vi "get channels.vi"(11 "module configuration in":refnum<class "PID Module configuration.lvclass">) -> (2 "channels":refnum<class "TBM channel.lvclass">[](array[class]), 3 "module configuration out":refnum<class "PID Module configuration.lvclass">)   [LabVIEW 2013, in "PID Module configuration.lvclass"]
doc: "Returns all channels used by a module."
uses:
  PID Module configuration.lvclass
  <vilib>/NI/Tag Bus Module Framework/module configuration/TBM module configuration.lvclass
  <vilib>/NI/Tag Bus Module Framework/channel/TBM channel.lvclass
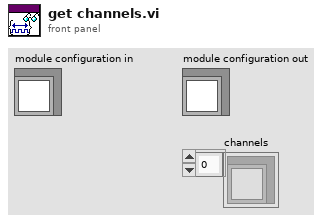
[diagram p1: front panel]
types:
  T1 = typedef "PID Module configuration.lvclass/PID array element.ctl" = cluster{"Loop ID":string, "Tags":cluster{"Setpoint":string, "Process Variable":string, "Output":string}, "Gains":cluster{"P":dbl, "I":dbl, "D":dbl}, "Range":cluster{"High":dbl, "Low":dbl}}
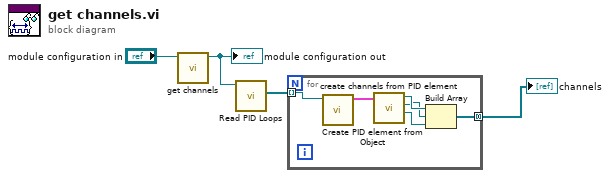
[diagram p0: block diagram]
diagram:
  n1 = call-parent "get channels.vi"("module configuration in"="module configuration in") -> ("module configuration out"=w3:refnum<class "PID Module configuration.lvclass">)  [unwired: 9 in, 1 out]
  "module configuration out" <- w3
  n2 = call-dynamic "Read PID Loops.vi"("Tagbus PID Module configuration in"=w3) -> ("PID Loops"=w2:refnum<class "PID Loop.lvclass">[])  [unwired: 8 in, 2 out]
  n3 = for {
    tunnel: w2 -> [w10] mode=indexing
    tunnel: [w5] -> w1 mode=concatenating
    n4 = call "Create PID element from Object.vi"("PID Loop in"=w10) -> ("line"=w9:T1)  [unwired: 10 in]
    n5 = call "create channels from PID element.vi"("line item in"=w9) -> ("Output Channel Out"=w7:refnum<class "TBM channel.lvclass">, "Process Variable Channel Out"=w6:refnum<class "TBM channel.lvclass">, "Setpoint Channel Out"=w8:refnum<class "TBM channel.lvclass">)  [unwired: 8 in]
    n6 = Build Array(w8, w6, w7) -> (w5:refnum<class "TBM channel.lvclass">[])
  }
  "channels" <- w1
